vi "LJUD UE9RAW CommConfig.vi"(7 "Comm Settings":T1={"Open LabJack "=TRUE, "Use USB"=TRUE, "IP Address"="192.168.1.209", "PortA"=52360, "PortB"=0}, 8 "error in (no error)":errorcluster, 10 "New Params":T2, 11 "Handle In":i32) -> (0 "error out":errorcluster, 1 "Ethernet Params":T4, 2 "Local ID":u8, 3 "Handle Out":i32, 4 "Other Params":T3 {"Comm Firmware Version" format="%.2f"; "Hardware Version" format="%.2f"})   [LabVIEW 2020]
panel:
  out "Write Array":u8[](array[numeric]) format="%.0x"
  out "Read Array":u8[](array[numeric]) format="%.0x"
  # "22"
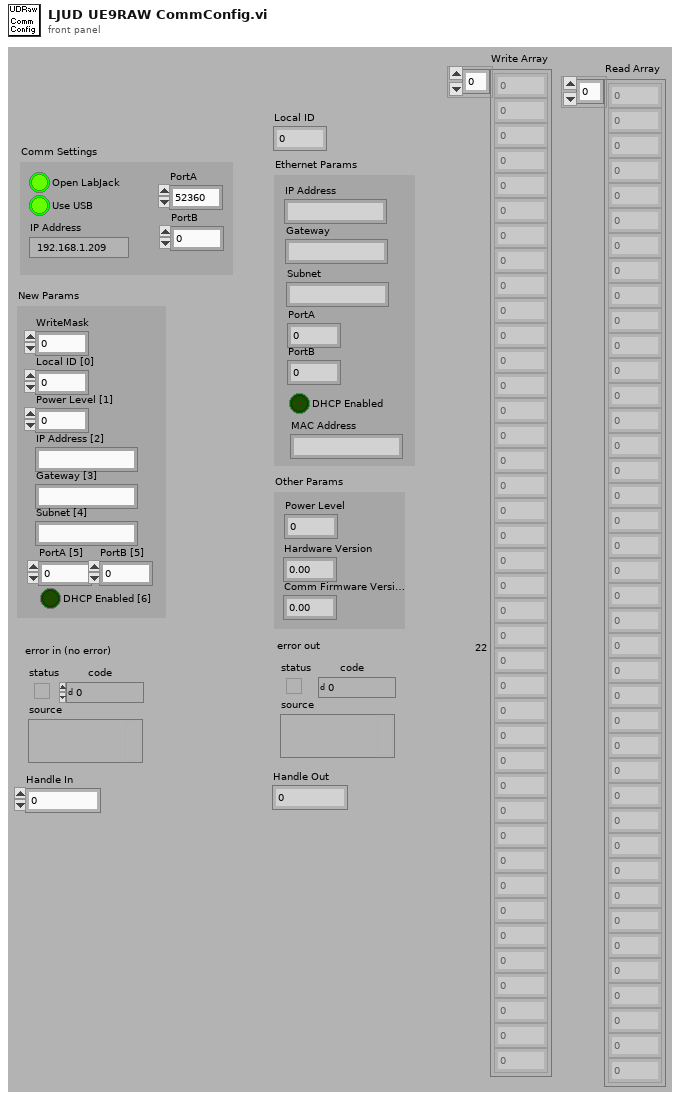
[diagram p1: front panel]
types:
  T1 = cluster{"Open LabJack ":bool, "Use USB":bool, "IP Address":string, "PortA":u16, "PortB":u16}
  T2 = cluster{"WriteMask":u8, "Local ID [0]":u8, "Power Level [1]":u8, "IP Address [2]":string, "Gateway [3]":string, "Subnet [4]":string, "PortA [5]":u16, "PortB [5]":u16, "DHCP Enabled [6]":bool}
  T3 = cluster{"Hardware Version":dbl, "Comm Firmware Version":dbl, "Power Level":u8}
  T4 = cluster{"IP Address":string, "PortA":u16, "PortB":u16, "Gateway":string, "Subnet":string, "DHCP Enabled":bool, "MAC Address":string}
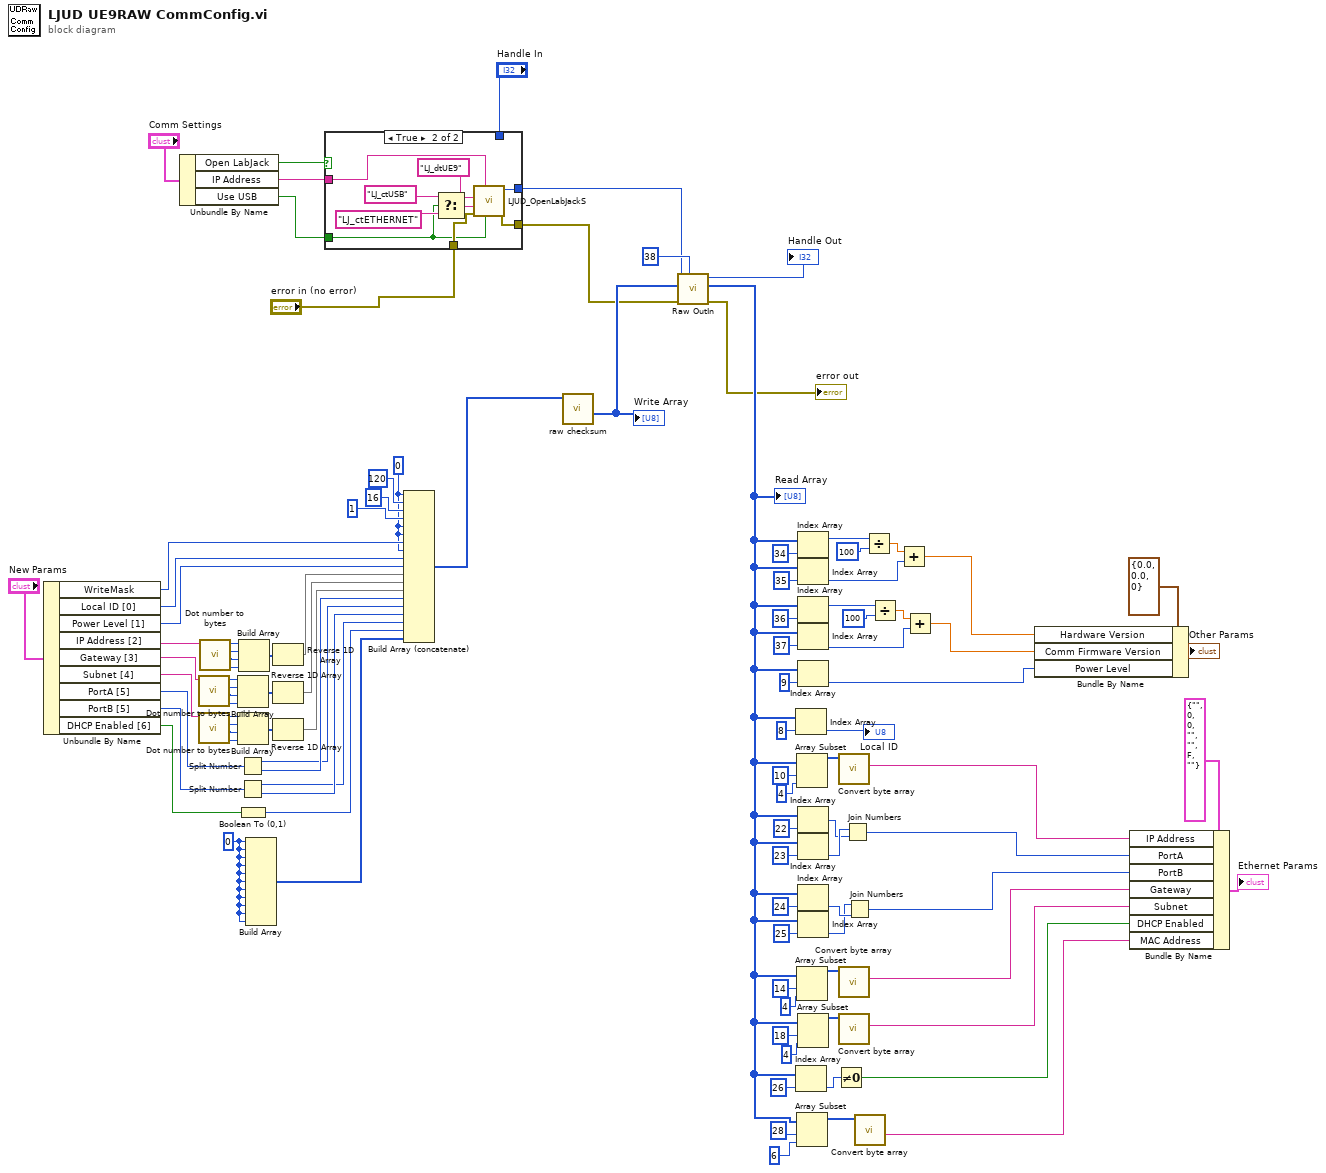
[diagram p0: block diagram]
diagram:
  w22 = u8 0 ("Input Element")
  w48 = u8 0 ("Input Element")
  n1 = Unbundle By Name("New Params") -> ("WriteMask"=w49:u8, "Local ID [0]"=w47:u8, "Power Level [1]"=w46:u8, "IP Address [2]"=w45:string, "Gateway [3]"=w32:string, "Subnet [4]"=w31:string, "PortA [5]"=w30:u16, "PortB [5]"=w29:u16, "DHCP Enabled [6]"=w24:bool)
  n2 = Unbundle By Name("Comm Settings") -> ("Open LabJack"=w1:bool, "IP Address"=w2:string, "Use USB"=w3:bool)
  n3 = call "Dot number to bytes.vi"("Dot # (Decimal String)"=w32) -> ("4th Byte"=w40:u8, "3rd Byte"=w39:u8, "2nd Byte"=w38:u8, "1st Byte (MSB)"=w37:u8)  [unwired: 4 in, 3 out]
  n4 = call "Dot number to bytes.vi"("Dot # (Decimal String)"=w31) -> ("4th Byte"=w33:u8, "3rd Byte"=w34:u8, "2nd Byte"=w35:u8, "1st Byte (MSB)"=w36:u8)  [unwired: 4 in, 3 out]
  n5 = call "Dot number to bytes.vi"("Dot # (Decimal String)"=w45) -> ("4th Byte"=w41:u8, "3rd Byte"=w42:u8, "2nd Byte"=w43:u8, "1st Byte (MSB)"=w44:u8)  [unwired: 4 in, 3 out]
  n6 = Build Array(w37, w38, w39, w40) -> (w18:u8[])
  n7 = Build Array(w36, w35, w34, w33) -> (w17:u8[])
  n8 = Split Number(x=w30) -> (hi(x)=w27:u8, lo(x)=w28:u8)
  n9 = Split Number(x=w29) -> (hi(x)=w25:u8, lo(x)=w26:u8)
  n10 = Boolean To (0,1)(Boolean=w24) -> (0, 1=w23:i16)
  n11 = Build Array(w44, w43, w42, w41) -> (w19:u8[])
  n12 = Build Array(w22, w22, w22, w22, w22, w22, w22, w22, w22, w22, w22) -> (w21:u8[])
  n13 = Reverse 1D Array(array=w19) -> (reversed array=w16:u8[])
  n14 = Reverse 1D Array(array=w18) -> (reversed array=w15:u8[])
  n15 = Reverse 1D Array(array=w17) -> (reversed array=w14:u8[])
  n16 = case shown="True" w1 {
    tunnel: w2 -> [_ w109]
    tunnel: "error in (no error)" -> [w106 w113]
    tunnel: [w106 w112] -> w5
    tunnel: [w105 w110] -> w6
    tunnel: w3 -> [_ w111]
    tunnel: "Handle In" -> [w105 _]
    frame False {
    }
    frame True {
      n17 = Select(t="LJ_ctUSB" ("ConnectionType"), s=w111, f="LJ_ctETHERNET" ("ConnectionType")) -> (s? t:f=w107:string)
      n18 = call "LJUD_OpenLabJackS.vi"("FirstFound"=w111, "Address"=w109, "error in"=w113, "ConnectionType"=w107, "DeviceType"="LJ_dtUE9") -> ("error out"=w112:errorcluster, "Handle"=w110:i32)  [unwired: 4 in, 1 out]
    }
  }
  n19 = Build Array (concatenate)(w48, u8 120 ("Input Element"), u8 16 ("Input Element"), u8 1 ("Input Element"), w48, w48, w49, w48, w47, w46, w16, w15, w14, w28, w27, w26, w25, w23, w21) -> (w20:i16[])
  n20 = call "raw checksum.vi"("Array"=w20) -> ("Array Output"=w13:u8[])  [unwired: 3 in, 7 out]
  "Write Array" <- w13
  n21 = call "Raw OutIn.vi"("# of bytes to read in"=38 ("# of bytes to read"), "error in"=w5, "Raw Out"=w13, "Handle In"=w6) -> ("error out"=→"error out":errorcluster, "Raw In"=w11:u8[], "Handle Out"=→"Handle Out":i32)  [unwired: 4 in, 1 out]
  "Read Array" <- w11
  n22 = Index Array(array=w11, index=8 ("Index")) -> (element=→"Local ID":u8)
  n23 = Index Array(array=w11, index=26 ("Index")) -> (element=w68:u8)
  n24 = Array Subset(array=w11, index=10 ("Index"), length=4 ("Array Length")) -> (w56:u8[])
  n25 = Array Subset(array=w11, index=14 ("Index"), length=4 ("Array Length")) -> (w60:u8[])
  n26 = Array Subset(array=w11, index=28 ("Index"), length=6 ("Array Length")) -> (w64:u8[])
  n27 = Index Array(array=w11, index=34 ("Index")) -> (element=w91:u8)
  n28 = Index Array(array=w11, index=35 ("Index")) -> (element=w88:u8)
  n29 = Index Array(array=w11, index=36 ("Index")) -> (element=w85:u8)
  n30 = Index Array(array=w11, index=37 ("Index")) -> (element=w84:u8)
  n31 = Index Array(array=w11, index=9 ("Index")) -> (element=w76:u8)
  n32 = Index Array(array=w11, index=22 ("Index")) -> (element=w82:u8)
  n33 = Index Array(array=w11, index=23 ("Index")) -> (element=w83:u8)
  n34 = Index Array(array=w11, index=24 ("Index")) -> (element=w81:u8)
  n35 = Index Array(array=w11, index=25 ("Index")) -> (element=w80:u8)
  n36 = Array Subset(array=w11, index=18 ("Index"), length=4 ("Array Length")) -> (w59:u8[])
  n37 = Not Equal To 0?(x=w68) -> (x != 0?=w67:bool)
  n38 = call "Convert byte array.vi"("Byte Array"=w56) -> ("Dot Decimal String"=w54:string)  [unwired: 7 in, 3 out]
  n39 = call "Convert byte array.vi"("Byte Array"=w60) -> ("Dot Decimal String"=w58:string)  [unwired: 7 in, 3 out]
  n40 = call "Convert byte array.vi"("Byte Array"=w59) -> ("Dot Decimal String"=w57:string)  [unwired: 7 in, 3 out]
  n41 = Join Numbers(hi=w83, lo=w82) -> ((hi.lo)=w71:u16)
  n42 = Join Numbers(hi=w80, lo=w81) -> ((hi.lo)=w70:u16)
  n43 = call "Convert byte array.vi"("Byte Array"=w64) -> ("Dot Hex String"=w63:string)  [unwired: 7 in, 3 out]
  n44 = Divide(x=w91, y=u8 100) -> (x/y=w89:dbl)
  n45 = Divide(x=w85, y=u8 100) -> (x/y=w87:dbl)
  n46 = Add(x=w89, y=w88) -> (x+y=w74:dbl)
  n47 = Add(x=w87, y=w84) -> (x+y=w75:dbl)
  n48 = Bundle By Name(cluster=T3 {"Hardware Version"=0.0, "Comm Firmware Version"=0.0, "Power Level"=0} ("Other Params"), "Hardware Version"=w74, "Comm Firmware Version"=w75, "Power Level"=w76) -> (→"Other Params":T3)
  n49 = Bundle By Name(cluster=T4 {"IP Address"="", "PortA"=0, "PortB"=0, "Gateway"="", "Subnet"="", "DHCP Enabled"=FALSE, "MAC Address"=""} ("Ethernet Params"), "IP Address"=w54, "PortA"=w71, "PortB"=w70, "Gateway"=w58, "Subnet"=w57, "DHCP Enabled"=w67, "MAC Address"=w63) -> (→"Ethernet Params":T4)
